vi "Variant_to_XML-Tag.vi"(5 "parameter":string, 7 "type info":string, 8 "error in (no error)":errorcluster, 11 "variant":variant) -> (0 "error out":errorcluster, 3 "XML tag":string)   [LabVIEW 2013]
doc: "Converts a variant, which contains an element or an array of elements of almost any data type, to an XML tag, where the input \"parameter\" is the name of the tag, \"type info\" is the attribute name plus its value (e.g. type=\"amplitude\") and the element value(s) of the variant is the content of the tag."
uses:
  <vilib>/Utility/VariantDataType/VariantType.lvlib
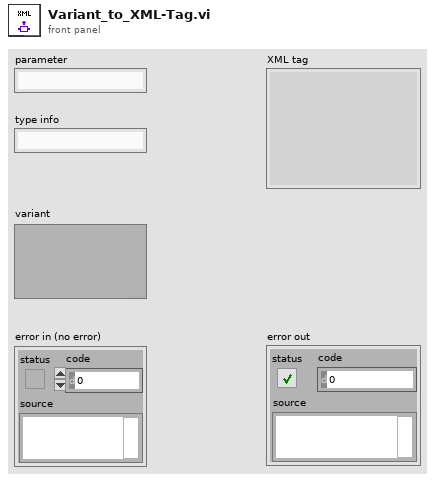
[diagram p1: front panel]
types:
  T1 = typedef "VariantType.lvlib/Type.ctl" = enum8{"Invalid Type", "Void", "I8", "I16", "I32", "I64", "U8", "U16", "U32", "U64", "Single Float", "Double Float", "Extended Float", "Single Complex", "Double Complex", "Extended Complex", "Enum U8", "Enum U16", "Enum U32", "Enum U64", "Single Float With Unit", "Double Float With Unit", "Extended Float With Unit", "Single Complex with Unit", "Double Complex with Unit", "Extended Complex with Unit", "Boolean", "String", "Path", "Picture", "Tag", "Array", "Cluster", "Variant", "LV Variant", "Waveform", "Timestamp", "Digital Waveform", "Digital Data", "ExpressData", "Refnum", "External Data", "VI", "Poly VI", "LabVIEW Class Instance", "Fixed Point"}
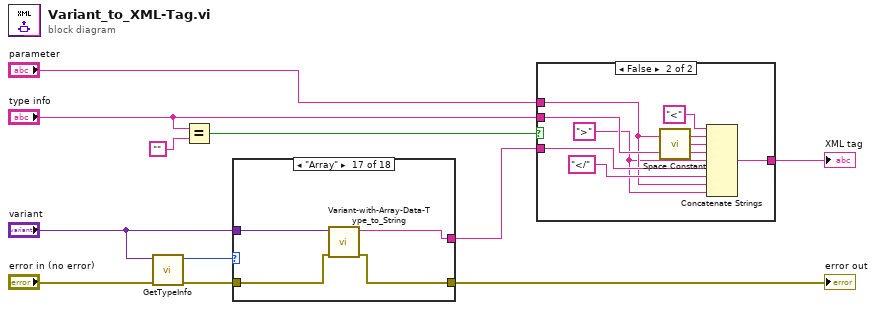
[diagram p0: block diagram]
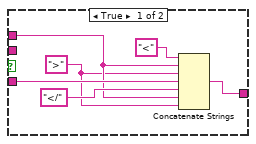
[diagram p2: hidden frame]
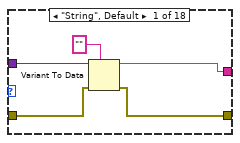
[diagram p3: hidden frame]
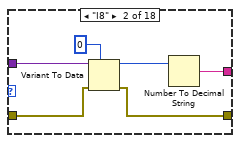
[diagram p4: hidden frame]
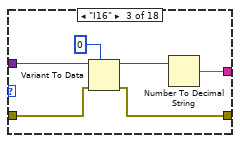
[diagram p5: hidden frame]
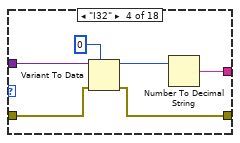
[diagram p6: hidden frame]
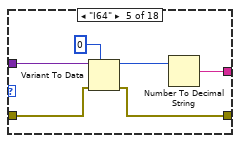
[diagram p7: hidden frame]
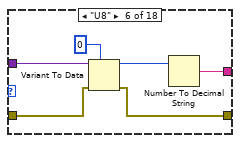
[diagram p8: hidden frame]
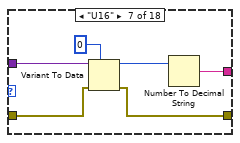
[diagram p9: hidden frame]
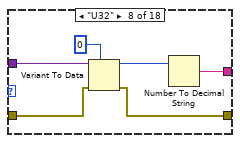
[diagram p10: hidden frame]
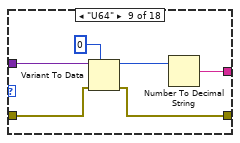
[diagram p11: hidden frame]
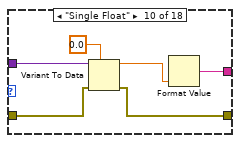
[diagram p12: hidden frame]
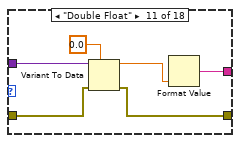
[diagram p13: hidden frame]
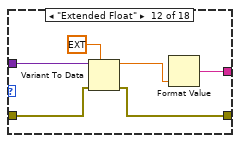
[diagram p14: hidden frame]
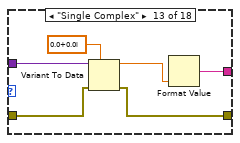
[diagram p15: hidden frame]
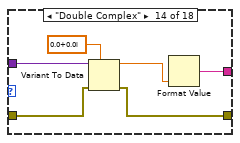
[diagram p16: hidden frame]
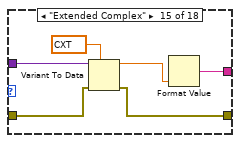
[diagram p17: hidden frame]
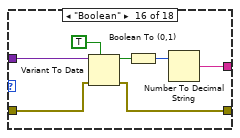
[diagram p18: hidden frame]
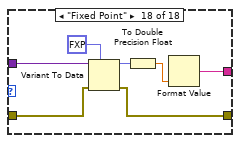
[diagram p19: hidden frame]
diagram:
  n1 = call <vilib>:"GetTypeInfo.vi"("error in (no error)"="error in (no error)", "Variant"="variant") -> ("error out"=w4:errorcluster, "Type Enum"=w11:T1)  [unwired: 5 in, 3 out]
  n2 = Equal?(x="type info", y="") -> (x = y?=w9:bool)
  n3 = case shown="\"Array\"" w11 {
    tunnel: "variant" -> [w16 w22 w28 w34 w40 w46 w52 w58 w64 w70 w76 w82 w88 w94 w100 w107 w111 w118]
    tunnel: [w12 w19 w25 w31 w37 w43 w49 w55 w61 w68 w74 w80 w86 w92 w98 w106 w108 w114] -> w7
    tunnel: w4 -> [w14 w17 w23 w29 w35 w41 w47 w53 w59 w66 w72 w78 w84 w90 w96 w104 w110 w115]
    tunnel: [w15 w18 w24 w30 w36 w42 w48 w54 w60 w67 w73 w79 w85 w91 w97 w105 w109 w116] -> w2
    frame "String", Default {
      n4 = Variant To Data(error in=w14, type="", Variant=w16) -> (data=w12:string, error out=w15:errorcluster)
    }
    frame "I8" {
      n5 = Variant To Data(error in=w17, type=i8 0, Variant=w22) -> (data=w21:i8, error out=w18:errorcluster)
      n6 = Number To Decimal String(number=w21) -> (decimal integer string=w19:string)  [unwired: 1 in]
    }
    frame "I16" {
      n7 = Variant To Data(error in=w23, type=i16 0, Variant=w28) -> (data=w27:i16, error out=w24:errorcluster)
      n8 = Number To Decimal String(number=w27) -> (decimal integer string=w25:string)  [unwired: 1 in]
    }
    frame "I32" {
      n9 = Variant To Data(error in=w29, type=0, Variant=w34) -> (data=w33:i32, error out=w30:errorcluster)
      n10 = Number To Decimal String(number=w33) -> (decimal integer string=w31:string)  [unwired: 1 in]
    }
    frame "I64" {
      n11 = Variant To Data(error in=w35, type=i64 0, Variant=w40) -> (data=w39:i64, error out=w36:errorcluster)
      n12 = Number To Decimal String(number=w39) -> (decimal integer string=w37:string)  [unwired: 1 in]
    }
    frame "U8" {
      n13 = Variant To Data(error in=w41, type=u8 0, Variant=w46) -> (data=w45:u8, error out=w42:errorcluster)
      n14 = Number To Decimal String(number=w45) -> (decimal integer string=w43:string)  [unwired: 1 in]
    }
    frame "U16" {
      n15 = Variant To Data(error in=w47, type=u16 0, Variant=w52) -> (data=w51:u16, error out=w48:errorcluster)
      n16 = Number To Decimal String(number=w51) -> (decimal integer string=w49:string)  [unwired: 1 in]
    }
    frame "U32" {
      n17 = Variant To Data(error in=w53, type=u32 0, Variant=w58) -> (data=w57:u32, error out=w54:errorcluster)
      n18 = Number To Decimal String(number=w57) -> (decimal integer string=w55:string)  [unwired: 1 in]
    }
    frame "U64" {
      n19 = Variant To Data(error in=w59, type=u64 0, Variant=w64) -> (data=w63:u64, error out=w60:errorcluster)
      n20 = Number To Decimal String(number=w63) -> (decimal integer string=w61:string)  [unwired: 1 in]
    }
    frame "Single Float" {
      n21 = Variant To Data(error in=w66, type=sgl 0.0, Variant=w70) -> (data=w65:sgl, error out=w67:errorcluster)
      n22 = Format Value(value (0)=w65) -> (output string=w68:string)  [unwired: 2 in]
    }
    frame "Double Float" {
      n23 = Variant To Data(error in=w72, type=0.0, Variant=w76) -> (data=w71:dbl, error out=w73:errorcluster)
      n24 = Format Value(value (0)=w71) -> (output string=w74:string)  [unwired: 2 in]
    }
    frame "Extended Float" {
      n25 = Variant To Data(error in=w78, type=ext 0.0, Variant=w82) -> (data=w77:ext, error out=w79:errorcluster)
      n26 = Format Value(value (0)=w77) -> (output string=w80:string)  [unwired: 2 in]
    }
    frame "Single Complex" {
      n27 = Variant To Data(error in=w84, type=csg 0.0+0.0i, Variant=w88) -> (data=w83:csg, error out=w85:errorcluster)
      n28 = Format Value(value (0)=w83) -> (output string=w86:string)  [unwired: 2 in]
    }
    frame "Double Complex" {
      n29 = Variant To Data(error in=w90, type=cdb 0.0+0.0i, Variant=w94) -> (data=w89:cdb, error out=w91:errorcluster)
      n30 = Format Value(value (0)=w89) -> (output string=w92:string)  [unwired: 2 in]
    }
    frame "Extended Complex" {
      n31 = Variant To Data(error in=w96, type=cxt 0.0+0.0i, Variant=w100) -> (data=w95:cxt, error out=w97:errorcluster)
      n32 = Format Value(value (0)=w95) -> (output string=w98:string)  [unwired: 2 in]
    }
    frame "Boolean" {
      n33 = Variant To Data(error in=w104, type=TRUE, Variant=w107) -> (data=w102:bool, error out=w105:errorcluster)
      n34 = Boolean To (0,1)(Boolean=w102) -> (0, 1=w101:i16)
      n35 = Number To Decimal String(number=w101) -> (decimal integer string=w106:string)  [unwired: 1 in]
    }
    frame "Array" {
      n36 = call "Variant-with-Array-Data-Type_to_String.vi"("error in (no error)"=w110, "variant"=w111) -> ("error out"=w109:errorcluster, "string"=w108:string)  [unwired: 8 in]
    }
    frame "Fixed Point" {
      n37 = Variant To Data(error in=w115, type=fxp<+/-,64,32> 0.0, Variant=w118) -> (data=w113:fxp<+/-,64,32>, error out=w116:errorcluster)
      n38 = To Double Precision Float(number=w113) -> (double precision float=w112:dbl)
      n39 = Format Value(value (0)=w112) -> (output string=w114:string)  [unwired: 2 in]
    }
  }
  "error out" <- w2
  n40 = case shown="False" w9 {
    tunnel: "parameter" -> [w121 w127]
    tunnel: w7 -> [w123 w129]
    tunnel: "type info" -> [_ w130]
    tunnel: [w119 w125] -> w3
    frame True {
      w120 = ">" ("string")
      n41 = Concatenate Strings("<" ("string"), w121, w120, w123, "</" ("string"), w121, w120) -> (w119:string)
    }
    frame False {
      w126 = ">" ("string")
      n42 = call <vilib>:"Space Constant.vi"() -> ("String"=w131:string)
      n43 = Concatenate Strings("<" ("string"), w127, w131, w130, w126, w129, "</" ("string"), w127, w126) -> (w125:string)
    }
  }
  "XML tag" <- w3
